vi "Method_Const.vi"(4 "Value":i64, 5 "Input A":refnum<class "Abs_I64 Integer.lvclass">) -> (1 "Result":T1)   [LabVIEW 2021, in "Subtract_I64.lvclass"]
uses:
  Subtract_I64.lvclass
  Abs_Types/I64 Integer/Abs_I64 Integer.lvclass
  C:/Program Files (x86)/National Instruments/LabVIEW 2021/vi.lib/TSA/Abstract Data Classes/Abs_Types/Numeric/Abs_Numeric.lvclass
  Abs Type.ctl
  C:/TSA/LV_Abstract/Source/Functions/Support/Function/Two Terminal/I64/AbsFunc_Two Term_I64.lvclass
  C:/Program Files (x86)/National Instruments/LabVIEW 2021/vi.lib/TSA/Abstract Data Classes/Abs_Types/I64 Integer/Abs_I64 Integer.lvclass
  Support/Function/Two Terminal/I64/AbsFunc_Two Term_I64.lvclass/AbsFunc_Two Term_I64.ctl
  Support/Function/Two Terminal/I64/Properties/Write Numeric A.vi
  Support/Function/Two Terminal/I64/Properties/Write Numeric B.vi
  Constants/Support/I64/Const_I64.lvclass
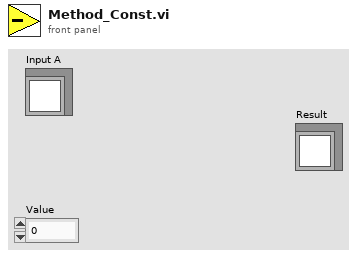
[diagram p1: front panel]
types:
  T1 = typedef "Subtract_I64.lvclass/Abs Type.ctl" = refnum<class "Abs_I64 Integer.lvclass">
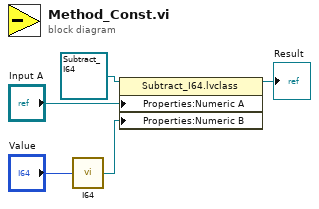
[diagram p0: block diagram]
diagram:
  n1 = call "I64.vi"("Value"="Value") -> ("Constant"=w2:refnum<class "Abs_I64 Integer.lvclass">)  [unwired: 4 in]
  n2 = property class="Subtract_I64.lvclass"(reference=refnum<class "Subtract_I64.lvclass"> refnum ("Subtract_DBL.lvclass"), "Properties:Numeric A"="Input A", "Properties:Numeric B"=w2) -> (reference out=→"Result":refnum<class "Subtract_I64.lvclass">)  [unwired: 1 in, 1 out]
